vi "DHE_WriteTP.vi"(5 "value":string, 6 "phys. unit":string, 7 "switches":string[](array[string]), 8 "error in (no error)":errorcluster, 9 "index in":i32, 10 "TP In":T1={"name"="", "type"="", "R_algor"=[], "board"="", "memory"="", "address"=0, "value"="", "Limits"={"upper"=0.0, "Lower"=0.0, "InRange"=FALSE, "nominal"=0.0}, "unit"="", "params"="", "permissions"="", "W_algor"=[], "description"="", "err_count"=0, "max_err"=3, "read"=FALSE, "lowrej"=0.0, "hirej"=0.0, "expupd"=FALSE} {"Limits"."nominal" format="%.2f"; "Limits"."Lower" format="%.2f"; "Limits"."upper" format="%.2f"}, 11 "refnum":i32) -> (0 "error out":errorcluster, 2 "response":string, 3 "refnum out":i32)   [LabVIEW 2016]
uses:
  DHE_TP.ctl
  DHE_TPLimits.ctl
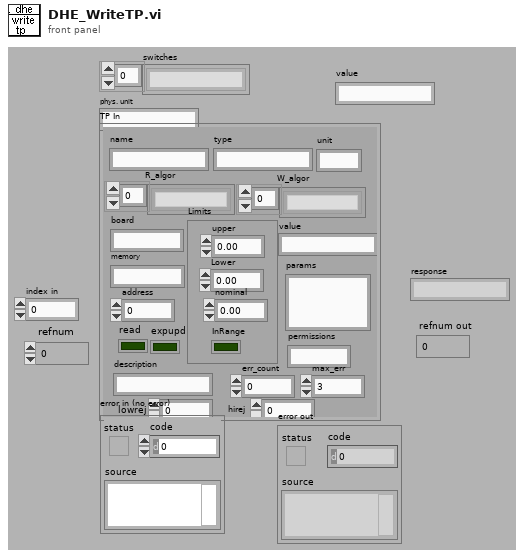
[diagram p1: front panel]
types:
  T1 = typedef "DHE_TP.ctl" = cluster{"name":string, "type":string, "R_algor":string[], "board":string, "memory":string, "address":i32, "value":string, "Limits":T2, "unit":string, "params":string, "permissions":string, "W_algor":string[], "description":string, "err_count":i32, "max_err":i32, "read":bool, "lowrej":dbl, "hirej":dbl, "expupd":bool}
  T2 = typedef "DHE_TPLimits.ctl" = cluster{"upper":dbl, "Lower":dbl, "InRange":bool, "nominal":dbl}
  T3 = enum16{"convert", "read from file", "get", "clear all", "get all"}
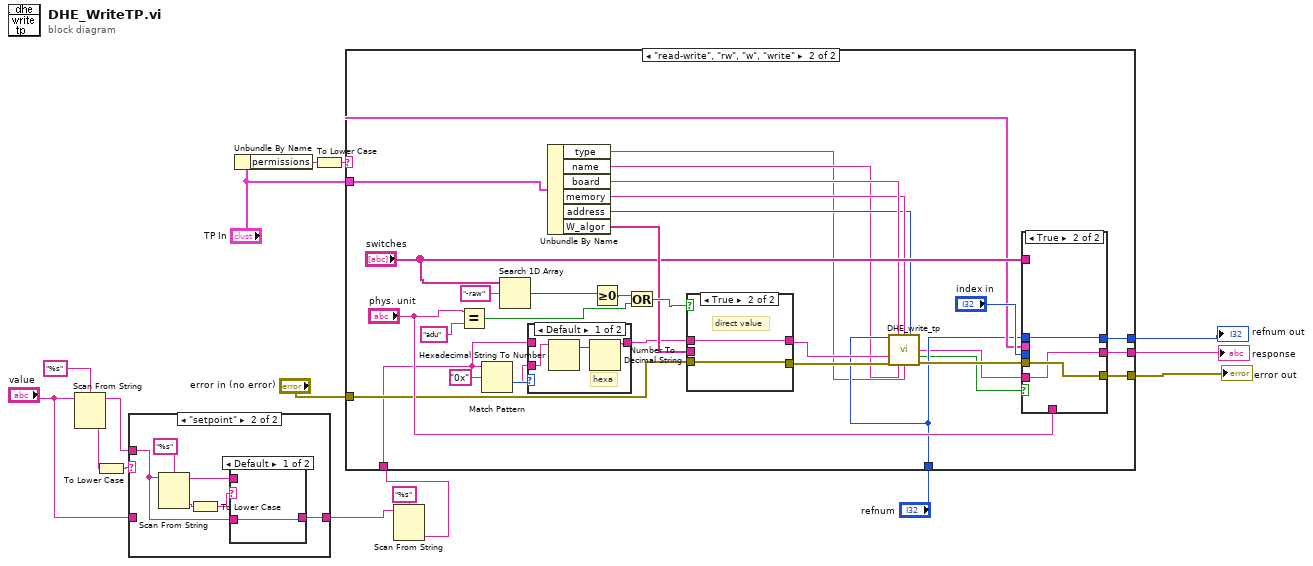
[diagram p0: block diagram]
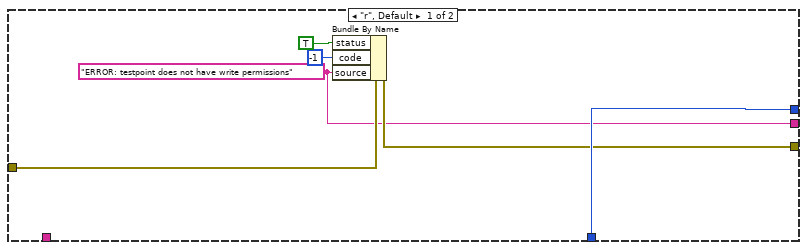
[diagram p4: hidden frame]
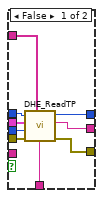
[diagram p5: hidden frame]
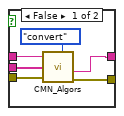
[diagram p7: hidden frame]
diagram:
  n1 = Scan From String(format string="%s", input string="value") -> (remaining string=w5:string, output 1=w7:string)  [unwired: 2 in, 3 out]
  n2 = To Lower Case(string=w7) -> (all lower case string=w6:string)
  n3 = case shown="\"setpoint\"" w6 {
    tunnel: w5 -> [_ w18]
    tunnel: "value" -> [w17 _]
    tunnel: [w17 w20] -> w3
    frame Default {
    }
    frame "setpoint" {
      n4 = Scan From String(format string="%s", input string=w18) -> (remaining string=w19:string, output 1=w22:string)  [unwired: 2 in, 3 out]
      n5 = To Lower Case(string=w22) -> (all lower case string=w21:string)
      n6 = case shown="Default" w21 {
        tunnel: [w24 w25] -> w20
        tunnel: w19 -> [_ w25]
        tunnel: w18 -> [w24 _]
        frame Default {
        }
        frame "value" {
        }
      }
    }
  }
  n7 = Unbundle By Name("TP In") -> ("permissions"=w12:string)
  n8 = To Lower Case(string=w12) -> (all lower case string=w11:string)
  n9 = Scan From String(format string="%s", input string=w3) -> (output 1=w1:string)  [unwired: 2 in, 4 out]
  n10 = case shown="\"read-write\", \"rw\", \"w\", \"write\"" w11 {
    tunnel: [w31 w52] -> w16
    tunnel: [w26 w51] -> w15
    tunnel: [w29 w50] -> w14
    tunnel: "TP In" -> [_ w49]
    tunnel: "error in (no error)" -> [w30 w48]
    tunnel: "refnum" -> [w31 w38]
    tunnel: w1 -> [_ w34]
    frame "r", Default {
      w26 = "ERROR: testpoint does not have write permissions" ("source")
      n11 = Bundle By Name(cluster=w30, "status"=TRUE, "code"=-1, "source"=w26) -> (w29:errorcluster)
    }
    frame "read-write", "rw", "w", "write" {
      n12 = Equal?(x="phys. unit", y="adu") -> (x = y?=w58:bool)
      n13 = Match Pattern(string=w34, regular expression="0x") -> (after substring=w44:string, offset past match=w46:i32)  [unwired: 3 out]
      n14 = Search 1D Array(1D array="switches", element="-raw") -> (index of element=w61:i32)  [unwired: 1 out]
      n15 = case shown="Default" w46 {
        tunnel: w34 -> [_ w78]
        tunnel: [w76 w78] -> w45
        tunnel: w44 -> [w75 _]
        frame Default {
          # "hexa"
          n16 = Hexadecimal String To Number(string=w75) -> (number=w77:u32)  [unwired: 3 out]
          n17 = Number To Decimal String(number=w77) -> (decimal integer string=w76:string)  [unwired: 1 out]
        }
        frame ..-1 {
          # "decimal"
        }
      }
      n18 = Unbundle By Name(w49) -> ("type"=w35:string, "name"=w36:string, "board"=w40:string, "memory"=w39:string, "address"=w37:i32, "W_algor"=w56:string[])
      n19 = Greater Or Equal To 0?(x=w61) -> (x >= 0?=w60:bool)
      n20 = Or(x=w60, y=w58) -> (x .or. y?=w57:bool)
      n21 = case shown="True" w57 {
        tunnel: w48 -> [w84 w86]
        tunnel: [w83 w86] -> w43
        tunnel: w56 -> [w81 _]
        tunnel: w45 -> [w80 w85]
        tunnel: [w79 w85] -> w41
        frame False {
          n22 = call "CMN_Algors.vi"("ValueIn"=w80, "algors"=w81, "error in (no error)"=w84, "action"=T3."convert") -> ("string value"=w79:string, "error out"=w83:errorcluster)  [unwired: 1 in, 4 out]
        }
        frame True {
          # "direct value"
        }
      }
      n23 = call "DHE_write_tp.vi"("fd"=w38, "board"=w40, "memory"=w39, "address"=w37, "value"=w41, "error in (no error)"=w43, "name"=w36, "type"=w35) -> ("return value"=w32:string, "busy"=w33:bool, "error out"=w42:errorcluster)  [unwired: 5 out]
      n24 = case shown="True" w33 {
        tunnel: "switches" -> [w71 _]
        tunnel: "phys. unit" -> [w70 _]
        tunnel: "index in" -> [w69 _]
        tunnel: [w68 w74] -> w52
        tunnel: [w67 w72] -> w51
        tunnel: [w66 w73] -> w50
        tunnel: w49 -> [w65 _]
        tunnel: w42 -> [w64 w73]
        tunnel: w38 -> [w63 w74]
        tunnel: w32 -> [_ w72]
        frame False {
          n25 = call "DHE_ReadTP.vi"("phys. unit"=w70, "switches"=w71, "error in (no error)"=w64, "index in"=w69, "TP In"=w65, "refnum"=w63) -> ("error out"=w66:errorcluster, "response"=w67:string, "refnum out"=w68:i32)  [unwired: 1 in, 2 out]
        }
        frame True {
        }
      }
    }
  }
  "refnum out" <- w16
  "response" <- w15
  "error out" <- w14
